vi "Myrio_4.vi"   [LabVIEW 2012]
uses:
  SubVIs/LVPresent_Globals.vi
panel:
  # "In order to connect the myRIO, you need to turn it on, and then a window  that looks like this one should pop up."
  # "Under hardware, you should select \"EvalRIO\" or \"myRIO\" depending on which version you are using,  and then you should put in the IP adress for your myRIO."
  # "When you have connected, the LED0 on you myRIO should turn on."
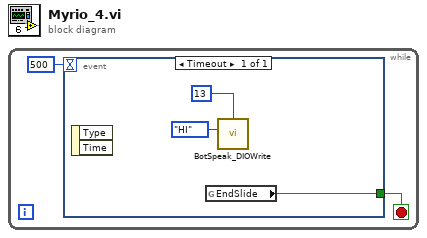
[diagram p0: block diagram]
diagram:
  n1 = while {
    stop <- w2 stop-if-true
    n2 = event shown="[0] Timeout" {
      selector: _ -> [_]
      dyn-events: _ -> [_]
      timeout: 500 -> [_]
      tunnel: [w5] -> w2
      event Timeout {
        n3 = event-data() -> ()  [unwired: 1 in, 2 out]
        n4 = global read "LVPresent_Globals.vi" "EndSlide"() -> (w5:bool)
        n5 = call <userlib>:"BotSpeak_DIOWrite.vi"("State"=enum32{"LO", "HI"}."HI", "DIO Line"=u32 13) -> ()  [unwired: 1 in, 2 out]
      }
    }
  }
